vi "Period Measurement.vi"() -> ()   [LabVIEW 2009]
uses:
  <vilib>/DAQmx/read.llb/DAQmx Read (Counter DBL 1Chan 1Samp).vi
  <vilib>/DAQmx/create/channels.llb/DAQmx Create Channel (CI-Period).vi
panel:
  in  "measurement time":dbl=0.001 format="%0.6f"
  in  "units":i32(ring)=10364 items=["Seconds"=10364, "Ticks"=10304, "From Custom Scale"=10065]
  in  "minimum value":dbl=1e-06 format="%.6f"
  in  "maximum value":dbl=0.1 format="%.6f"
  out "Period Measurement":dbl format="%.3f"
  in  "starting edge":i32(ring)=10280 items=["Rising"=10280, "Falling"=10171]
  in  "counter":tag
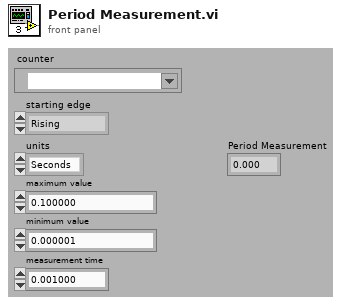
[diagram p1: front panel]
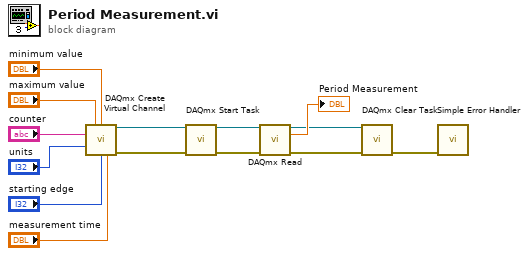
[diagram p0: block diagram]
diagram:
  n1 = call-poly <vilib>:"DAQmx Create Virtual Channel.vi"("maximum value"="maximum value", "minimum value"="minimum value", "counter"="counter", "units"="units", "starting edge"="starting edge", "measurement time"="measurement time") -> ("task out"=w10:refnum<k21>, "error out"=w8:errorcluster)  [unwired: 8 in]
  n2 = call <vilib>:"DAQmx Start Task.vi"("task/channels in"=w10, "error in"=w8) -> ("task out"=w9:refnum<k21>, "error out"=w7:errorcluster)  [unwired: 12 in]
  n3 = call-poly <vilib>:"DAQmx Read.vi"("task/channels in"=w9, "error in"=w7) -> ("task out"=w6:refnum<k21>, "data"=→"Period Measurement":dbl, "error out"=w5:errorcluster)  [unwired: 11 in]
  n4 = call <vilib>:"DAQmx Clear Task.vi"("task in"=w6, "error in"=w5) -> ("error out"=w4:errorcluster)  [unwired: 13 in]
  n5 = call <vilib>:"Simple Error Handler.vi"("error in (no error)"=w4) -> ()  [unwired: 4 in, 5 out]
